vi "Configure External Modulation Source (Frequency Shift-Keying).vi"(6 "Range (5.0 Volts)":dbl(ring) items=["2.5", "5.0"], 7 "Level (2.5 Volts)":dbl, 8 "error in (no error)":errorcluster, 9 "Impedance (10000.0 Ohms)":dbl(ring) items=["50.0", "10000.0"], 10 "Channel (1: Channel1)":i32(ring) items=["Channel1", "Channel2"], 11 "VISA resource name":refnum<visa-resource-name>) -> (0 "error out":errorcluster, 3 "VISA resource name out":refnum<visa-resource-name>)   [LabVIEW 2009, in "Agilent 81150.lvlib"]
doc: "Configures external FSK modulation source (impedance, range and level) of the function generator."
uses:
  Agilent 81150.lvlib
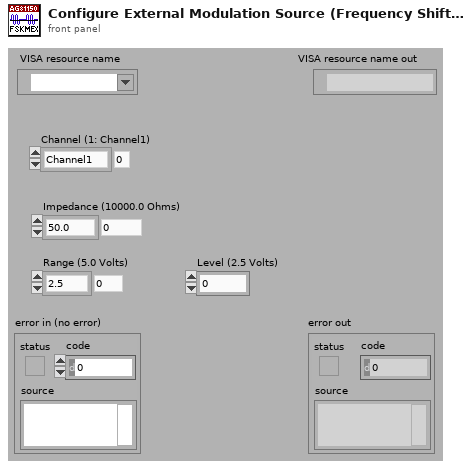
[diagram p1: front panel]
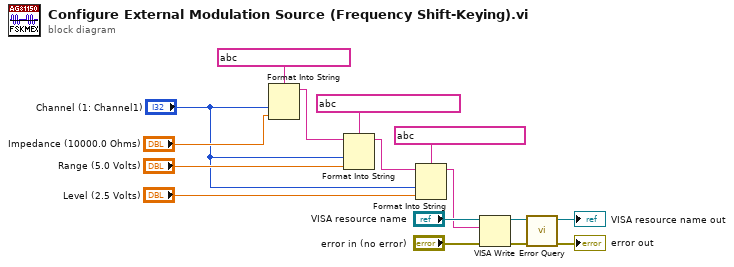
[diagram p0: block diagram]
diagram:
  n1 = Format Into String(format string=string ?, "Channel (1: Channel1)", "Impedance (10000.0 Ohms)") -> (resulting string=w10:string)  [unwired: 2 in, 1 out]
  n2 = Format Into String(format string=string ?, initial string=w10, "Channel (1: Channel1)", "Range (5.0 Volts)") -> (resulting string=w5:string)  [unwired: 1 in, 1 out]
  n3 = Format Into String(format string=string ?, initial string=w5, "Channel (1: Channel1)", "Level (2.5 Volts)") -> (resulting string=w4:string)  [unwired: 1 in, 1 out]
  n4 = VISA Write(VISA resource name="VISA resource name", write buffer=w4, error in (no error)="error in (no error)") -> (VISA resource name out=w12:refnum<visa-resource-name>, error out=w11:errorcluster)  [unwired: 1 out]
  n5 = call "Error Query.vi"("error in (no error)"=w11, "VISA resource name"=w12) -> ("error out"=→"error out":errorcluster, "VISA resource name out"=→"VISA resource name out":refnum<visa-resource-name>)  [unwired: 8 out]
